vi "BLM Move.vi"(4 "Mode IS:":bool, 5 "Steps/rot":dbl=8000.0, 6 "error in (no error)":errorcluster, 7 "Position / Distance":dbl=1.0 min=-193273528.32 max=193273528.0 step=0.09 format="%.2f", 8 "Motor Address":string="0", 9 "Port Address":refnum<visa-resource-name>) -> (0 "error out":errorcluster, 3 "Port Address Out":refnum<visa-resource-name>)   [LabVIEW 2024]
panel:
  out "Command string":string
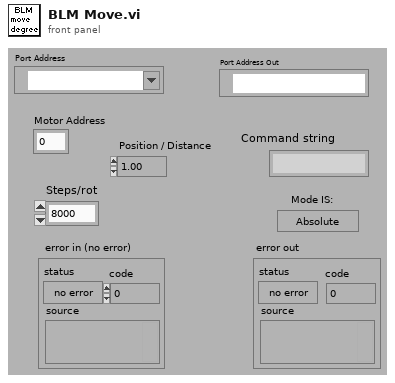
[diagram p1: front panel]
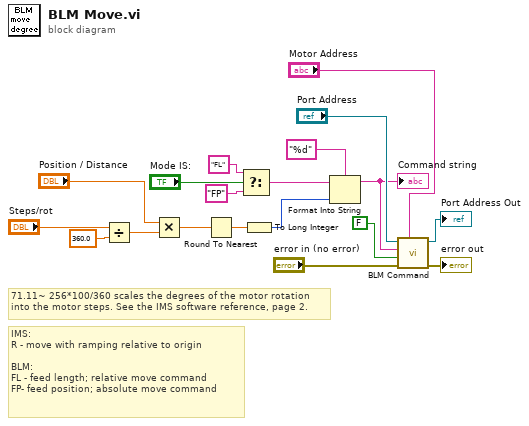
[diagram p0: block diagram]
diagram:
  # "IMS:\nR - move with ramping relative to origin\n\nBLM:\nFL - feed length; relative move command\nFP- feed position; absolute move command"
  # "71.11~ 256*100/360 scales the degrees of the motor rotation\ninto the motor steps. See the IMS software reference, page 2."
  n1 = Divide(x="Steps/rot", y=360.0) -> (x/y=w7:dbl)
  n2 = Multiply(x="Position / Distance", y=w7) -> (x*y=w17:dbl)
  n3 = Round To Nearest(number=w17) -> (nearest integer value=w16:dbl)
  n4 = Select(t="FL", s="Mode IS:", f="FP") -> (s? t:f=w11:string)
  n5 = To Long Integer(number=w16) -> (32bit integer=w8:i32)
  n6 = Format Into String(format string="%d", initial string=w11, w8) -> (resulting string=w10:string)  [unwired: 1 in, 1 out]
  "Command string" <- w10
  n7 = call "BLM Command.vi"("Motor Address"="Motor Address", "error in (no error)"="error in (no error)", "Read Echo?"=FALSE, "Command"=w10, "Port Address"="Port Address") -> ("error out"=→"error out":errorcluster, "Port Address Out"=→"Port Address Out":refnum<visa-resource-name>)  [unwired: 1 in, 3 out]
